vi "getDeviceChannelSafeValues.vi"(8 "error in (no error)":errorcluster, 10 "device_name":string, 11 "deviceDataBase in":refnum<class "deviceDataBase.lvclass">) -> (0 "error out":errorcluster, 1 "SafeVaues":dbl[](array[numeric]), 2 "ChannelAddresses":string[](array[string]), 3 "deviceDataBase out":refnum<class "deviceDataBase.lvclass">)   [LabVIEW 2009, in "Tools.lvlib" / "DatabaseHelpers.lvlib" / "deviceDataBase.lvclass"]
uses:
  deviceDataBase.lvclass
  deviceDataBase.lvclass/deviceDataBase.ctl
  Database Objects/DeviceArray/DeviceArray.lvclass
  Database Objects/ChannelArray/ChannelArray.lvclass
  Database Objects/Channel/Channel.lvclass
  Database Objects/device/device.lvclass
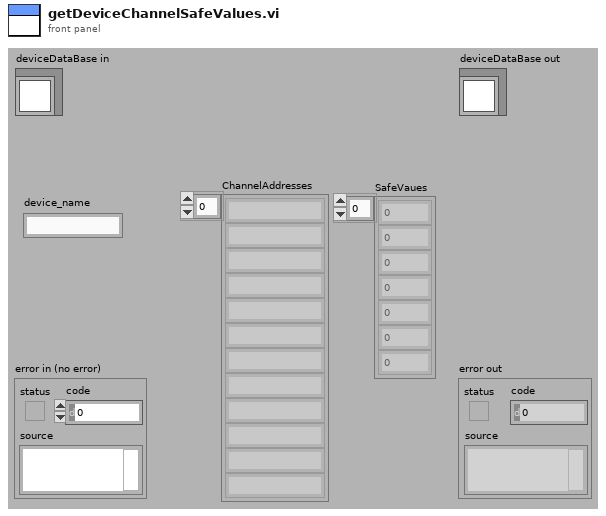
[diagram p1: front panel]
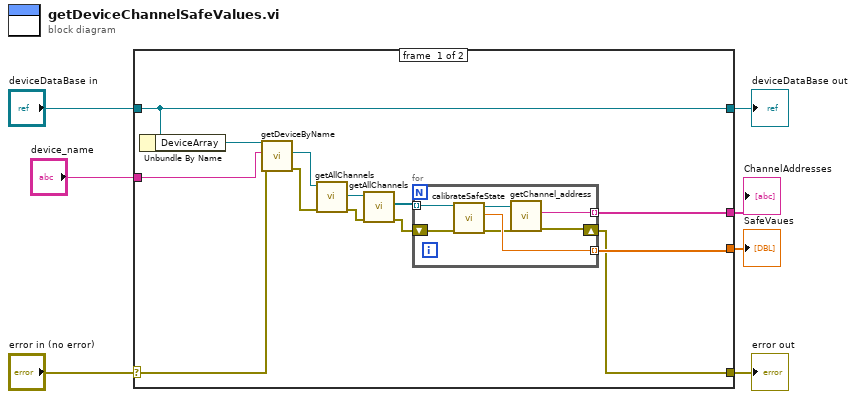
[diagram p0: block diagram]
diagram:
  n1 = case shown="No Error" "error in (no error)" {
    selector: "error in (no error)" -> [w17 w29]
    tunnel: [w12 w29] -> w6
    tunnel: [w20 w28] -> w4
    tunnel: "deviceDataBase in" -> [w20 w28]
    tunnel: "device_name" -> [w18 _]
    tunnel: [w14 _] -> w1
    tunnel: [w13 _] -> w2
    frame #0 {
      n2 = Unbundle By Name(w20) -> ("DeviceArray"=w19:refnum<class "DeviceArray.lvclass">)
      n3 = call "getDeviceByName.vi"("error in (no error)"=w17, "deviceName"=w18, "DeviceArray in"=w19) -> ("error out"=w8:errorcluster, "device.lvclass"=w9:refnum<class "device.lvclass">)  [unwired: 5 in, 2 out]
      n4 = call "getAllChannels.vi"("error in (no error)"=w8, "device in"=w9) -> ("error out"=w11:errorcluster, "ChannelArray"=w10:refnum<class "ChannelArray.lvclass">)  [unwired: 7 in, 1 out]
      n5 = call "getAllChannels.vi"("error in (no error)"=w11, "ChannelArray.lvclass in"=w10) -> ("error out"=w16:errorcluster, "channels"=w15:refnum<class "Channel.lvclass">[])  [unwired: 7 in, 1 out]
      n6 = for {
        shift-right: [w21] -> w12
        shift-left: w16 -> [w27]
        tunnel: w15 -> [w26] mode=indexing
        tunnel: [w25] -> w13 mode=indexing
        tunnel: [w22] -> w14 mode=indexing
        n7 = call "calibrateSafeState.vi"("error in (no error)"=w27, "Channel in"=w26) -> ("error out"=w23:errorcluster, "calibratedValue"=w25:dbl, "Channel out"=w24:refnum<class "Channel.lvclass">)  [unwired: 7 in]
        n8 = call "getChannel_address.vi"("error in (no error)"=w23, "Channel.lvclass in"=w24) -> ("error out"=w21:errorcluster, "channel_address"=w22:string)  [unwired: 7 in, 1 out]
      }
    }
    frame #1 {
    }
  }
  "error out" <- w6
  "deviceDataBase out" <- w4
  "SafeVaues" <- w2
  "ChannelAddresses" <- w1
